vi "FTW-ProjectManager-GetProjectOwningApplicationRef.vi"(0 "Project Manager":refnum<class "FTW-ProjectManager.lvclass">, 11 "error in":errorcluster) -> (4 "Project Manager out":refnum<class "FTW-ProjectManager.lvclass">, 6 "Application":refnum<vi>, 8 "App Name":string, 10 "Context Name":string, 15 "error out":errorcluster)   [LabVIEW 2012, in "FTW-ProjectManager.lvclass"]
uses:
  FTW-ProjectManager.lvclass
  FTW-ProjectManager.lvclass/FTW-ProjectManager.ctl
panel:
  # "Inputs"
  # "Outputs"
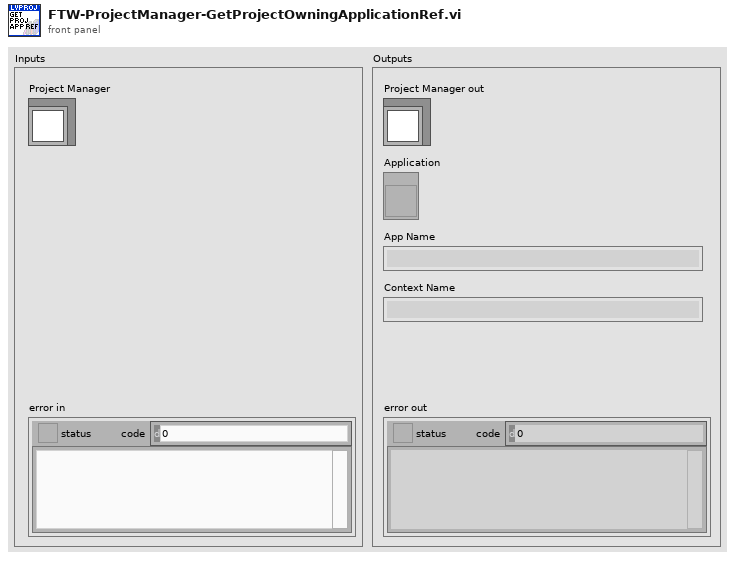
[diagram p1: front panel]
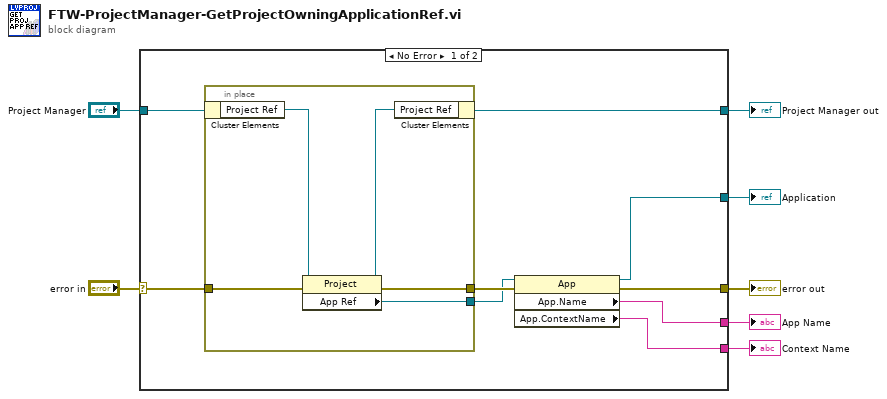
[diagram p0: block diagram]
diagram:
  n1 = case shown="No Error" "error in" {
    selector: "error in" -> [w16 w23]
    tunnel: [w13 w23] -> w7
    tunnel: [w8 w22] -> w5
    tunnel: "Project Manager" -> [w9 w22]
    tunnel: [w11 _] -> w3
    tunnel: [w15 _] -> w2
    tunnel: [w10 _] -> w1
    frame No Error {
      n2 = in-place {
        in-place-border: w16 -> [w21]
        in-place-border: [w20] -> w14
        in-place-border: [w19] -> w12
        n3 = in-place-cluster #1(w9) -> ("Project Ref"=w18:refnum<vi>)
        n4 = property class="Project"(reference=w18, error in=w21) -> (reference out=w17:refnum<vi>, error out=w20:errorcluster, "App Ref"=w19:refnum<vi>)
        n5 = in-place-cluster #1("Project Ref"=w17) -> (w8:refnum<class "FTW-ProjectManager.lvclass">)
      }
      n6 = property class="App"(reference=w12, error in=w14) -> (reference out=w11:refnum<vi>, error out=w13:errorcluster, "App.Name"=w15:string, "App.ContextName"=w10:string)
    }
    frame Error {
    }
  }
  "error out" <- w7
  "Project Manager out" <- w5
  "Application" <- w3
  "App Name" <- w2
  "Context Name" <- w1
